vi "Is Error.vi"(11 "Base Queue in":refnum<class "Base Queue.lvclass">) -> (3 "Base Queue out":refnum<class "Base Queue.lvclass">)   [LabVIEW 2021, in "jettl.lvlib" / "Base Queue.lvlib" / "Base Queue.lvclass"]
uses:
  Base Queue.lvclass
  State/Error State/Error State.lvclass
  C:/git/jettl/src/jettl/Base Queue/State/State/State.lvclass
  Base Queue.lvclass/Base Queue.ctl
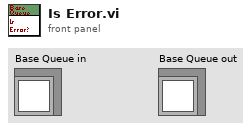
[diagram p1: front panel]
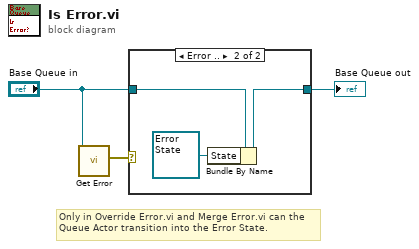
[diagram p0: block diagram]
diagram:
  # "Only in Override Error.vi and Merge Error.vi can the Queue Actor transition into the Error State."
  n1 = call-dynamic "Get Error.vi"("Base Queue in"="Base Queue in") -> ("Error"=w3:errorcluster)  [unwired: 10 in]
  n2 = case shown="Error .." w3 {
    tunnel: [w4 w6] -> w1
    tunnel: "Base Queue in" -> [w4 w7]
    frame No Error {
    }
    frame Error {
      n3 = Bundle By Name(cluster=w7, "State"=refnum<class "Error State.lvclass"> refnum ("jettl.lvlib:jettl Queue Actor.lvlib:Error State.lvclass")) -> (w6:refnum<class "Base Queue.lvclass">)
    }
  }
  "Base Queue out" <- w1
